vi "Agilent N6700 Series Data Log Voltage Sine Wave.vi"() -> ()   [LabVIEW 2018]
doc: "Configures the channel output range, waveform characteristics, sine wave, waveform trigger source, voltage trigger mode and enable output on a specified channel. This VI also configure the data logger, initiates data log, send a software trigger, configure data log markers and fetchs the peak to peak value of the data log.\n\n<b>Note:</b>\n\nThis VI only applies to the N6705B and N6705C DC Power Analyzer."
uses:
  Public/Configuration/Waveform/Configure Waveform (Sine Wave).vi
  <instrlib>/Agilent N6700 Series/Agilent N6700 Series.lvlib
panel:
  in  "Frequency (1.0 Hz)":dbl=1.0 format="%^.3e"
  in  "Data Log File Path":string="dlog example.dlog"
  in  "Voltage Range (5.0 V)":dbl=5.0 format="%^.3e"
  in  "Data Log Duration (15 s)":i32=15
  in  "Data Log Marker 2 (10.0 s)":dbl=10.0 format="%^.3e"
  in  "Data Log Marker 1 (7.5 s)":dbl=7.5 format="%^.3e"
  out "Peak to Peak Voltage":dbl format="%^.3e"
  in  "Channel Name (1)":string="1"
  in  "VISA resource name":refnum<visa-resource-name>
  # "(c) 2012-2019  National Instruments.  ALL RIGHTS RESERVED."
  # "Agilent N6705 DC Power Supply"
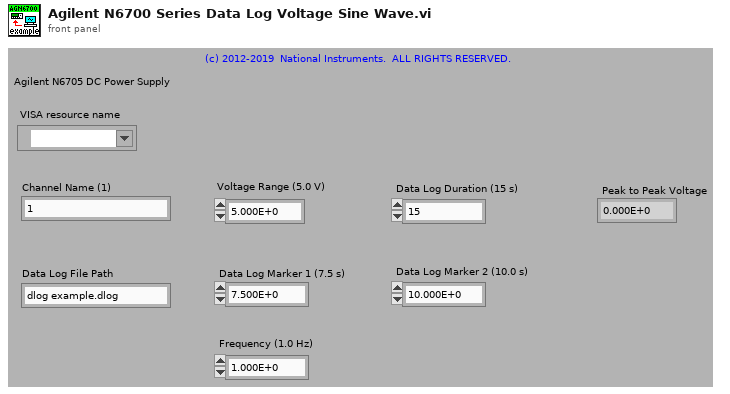
[diagram p1: front panel]
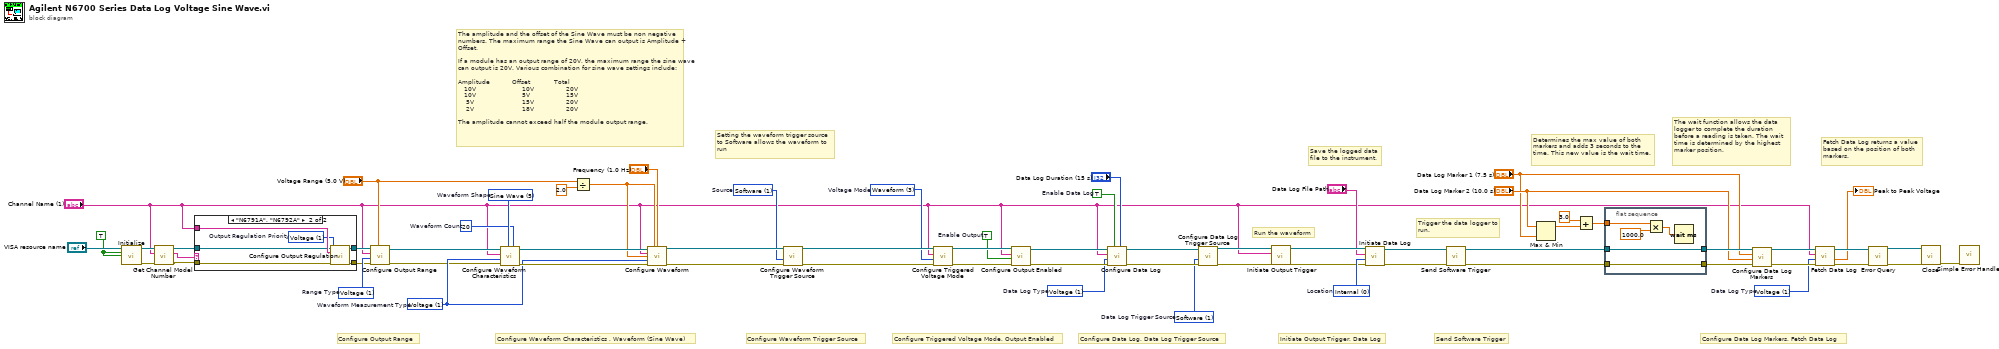
[diagram p0: block diagram]
diagram:
  w12 = 1 items=["Voltage"=1, "Current"=0]  # Data Log Type
  w25 = 20  # Waveform Count
  w26 = 1 items=["External", "Software", "Immediate", "Voltage1", "Voltage2", "Voltage3", "Voltage4", "Current1", "Current2", "Current3", "Current4"]  # Data Log Trigger Source
  w30 = 1 items=["Voltage"=1, "Current"=0]  # Range Type
  w37 = 3 items=["Fixed", "Step", "List", "Waveform"]  # Voltage Mode
  w11 = TRUE  # Enable Data Log
  w46 = TRUE  # Enable Output
  w51 = u16 1 items=["External", "Software", "Pin 1", "Pin 2", "Pin 3", "Transient 1", "Transient 2", "Transient 3", "Transient 4"]  # Source
  w38 = 1 items=["Voltage"=1, "Current"=0]  # Data Log Type
  w54 = TRUE ("Reset? (T: Yes)")
  w56 = 5 items=["None", "Constant Dwell", "Exponential", "Pulse", "Ramp", "Sine Wave", "Staircase", "Step", "Trapezoid", "Sequence", "User Defined"]  # Waveform Shape
  w57 = 0 items=["Internal", "External"]  # Location
  w58 = 1 items=["Voltage"=1, "Current"=0]  # Waveform Measurement Type
  # "Fetch Data Log returns a value\nbased on the position of both\nmarkers."
  # "Initiate Output Trigger, Data Log"
  # "Send Software Trigger"
  # "Configure Data Log Markers, Fetch Data Log"
  # "Configure Triggered Voltage Mode, Output Enabled"
  # "Configure Waveform Trigger Source"
  # "Run the waveform"
  # "Configure Output Range"
  # "Configure Data Log, Data Log Trigger Source"
  # "Configure Waveform Characteristics , Waveform (Sine Wave)"
  # "Determines the max value of both markers and adds 3 seconds to the time. This new value is the wait time."
  # "Trigger the data logger to run."
  # "Save the logged data\nfile to the instrument."
  # "Setting the waveform trigger source\nto Software allows the waveform to\nrun"
  # "The amplitude and the offset of the Sine Wave must be non negative numbers. The maximum range the Sine Wave can output is Amplitude + Offset.\n\nIf a module has an output range of 20V, the maximum range the sine wave can output is 20V. Various combination for sine wave settings include:\n\nAmplitude           Offset            Total\n   10V                       10V                20V\n   10V                       5V                  15V\n    5V                        15V                20V\n    2V                        18V                20V\n\nThe amplitude cannot exceed half the module output range."
  # "The wait function allows the data logger to complete the duration before a reading is taken. The wait\ntime is determined by the highest marker position."
  n1 = call "Initialize.vi"("VISA resource name"="VISA resource name", "ID Query? (T: Yes)"=w54, "Reset? (T: Yes)"=w54) -> ("VISA resource name out"=w6:refnum<visa-resource-name>, "error out"=w5:errorcluster)  [unwired: 11 in]
  n2 = call "Get Channel Model Number.vi"("error in (no error)"=w5, "Channel Name (1)"="Channel Name (1)", "VISA resource name"=w6) -> ("error out"=w4:errorcluster, "Model Number"=w2:string, "VISA resource name out"=w3:refnum<visa-resource-name>)  [unwired: 6 in]
  n3 = case shown="\"N6791A\", \"N6792A\"" w2 {
    tunnel: [w67 w73] -> w8
    tunnel: [w66 w72] -> w7
    tunnel: "Channel Name (1)" -> [_ w71]
    tunnel: w4 -> [w66 w68]
    tunnel: w3 -> [w67 w69]
    frame Default {
      # "The default priority for N679x is current."
    }
    frame "N6791A", "N6792A" {
      w70 = 1 items=["Voltage"=1, "Current"=0]  # Output Regulation Priority
      n4 = call "Configure Output Regulation.vi"("VISA resource name"=w69, "Channel Name (1)"=w71, "Output Regulation Priority (1: Voltage)"=w70, "error in (no error)"=w68) -> ("VISA resource name out"=w73:refnum<visa-resource-name>, "error out"=w72:errorcluster)  [unwired: 10 in]
    }
  }
  n5 = call "Configure Output Range.vi"("Range (0.0)"="Voltage Range (5.0 V)", "error in (no error)"=w7, "Range Type (1: Voltage)"=w30, "Channel Name (1)"="Channel Name (1)", "VISA resource name"=w8) -> ("error out"=w32:errorcluster, "VISA resource name out"=w31:refnum<visa-resource-name>)  [unwired: 5 in]
  n6 = call "Configure Waveform Characteristics.vi"("Waveform Count (1)"=w25, "Waveform Shape (0: None)"=w56, "error in (no error)"=w32, "Waveform Type (1: Voltage)"=w58, "Channel Name (1)"="Channel Name (1)", "VISA resource name"=w31) -> ("error out"=w59:errorcluster, "VISA resource name out"=w60:refnum<visa-resource-name>)  [unwired: 4 in]
  n7 = Divide(x="Voltage Range (5.0 V)", y=2.0) -> (x/y=w28:dbl)
  n8 = call-poly "Configure Waveform.vi"("VISA resource name"=w60, "Offset (0.0)"=w28, "Frequency (1.0 Hz)"="Frequency (1.0 Hz)", "Channel Name (1)"="Channel Name (1)", "Amplitude (0.0)"=w28, "Waveform Type (1: Voltage)"=w58, "error in (no error)"=w59) -> ("VISA resource name out"=w52:refnum<visa-resource-name>, "error out"=w53:errorcluster)  [unwired: 7 in]
  n9 = call "Configure Waveform Trigger Source.vi"("error in (no error)"=w53, "Source (2: Immediate)"=w51, "VISA resource name"=w52) -> ("error out"=w50:errorcluster, "VISA resource name out"=w49:refnum<visa-resource-name>)  [unwired: 7 in]
  n10 = call "Configure Triggered Voltage Mode.vi"("error in (no error)"=w50, "Voltage Mode (0: Fixed)"=w37, "Channel Name (1)"="Channel Name (1)", "VISA resource name"=w49) -> ("error out"=w47:errorcluster, "VISA resource name out"=w48:refnum<visa-resource-name>)  [unwired: 6 in]
  n11 = call "Configure Output Enabled.vi"("error in (no error)"=w47, "Enable Output (False)"=w46, "Channel Name (1)"="Channel Name (1)", "VISA resource name"=w48) -> ("error out"=w42:errorcluster, "VISA resource name out"=w41:refnum<visa-resource-name>)  [unwired: 6 in]
  n12 = call "Configure Data Log.vi"("Data Log Duration (30 s)"="Data Log Duration (15 s)", "Enable Data Log (True)"=w11, "error in (no error)"=w42, "Data Log Type (1: Voltage)"=w38, "Channel Name (1)"="Channel Name (1)", "VISA resource name"=w41) -> ("error out"=w39:errorcluster, "VISA resource name out"=w40:refnum<visa-resource-name>)  [unwired: 4 in]
  n13 = call "Configure Data Log Trigger Source.vi"("error in (no error)"=w39, "Data Log Trigger Source (2: Immediate)"=w26, "VISA resource name"=w40) -> ("error out"=w22:errorcluster, "VISA resource name out"=w24:refnum<visa-resource-name>)  [unwired: 7 in]
  n14 = call "Initiate Output Trigger.vi"("error in (no error)"=w22, "Channel Name (1)"="Channel Name (1)", "VISA resource name"=w24) -> ("error out"=w21:errorcluster, "VISA resource name out"=w23:refnum<visa-resource-name>)  [unwired: 7 in]
  n15 = call "Initiate Data Log.vi"("error in (no error)"=w21, "Location (0: Internal)"=w57, "Data Log File Path (data1.dlog)"="Data Log File Path", "VISA resource name"=w23) -> ("error out"=w35:errorcluster, "VISA resource name out"=w36:refnum<visa-resource-name>)  [unwired: 6 in]
  n16 = call "Send Software Trigger.vi"("error in (no error)"=w35, "VISA resource name"=w36) -> ("error out"=w34:errorcluster, "VISA resource name out"=w33:refnum<visa-resource-name>)  [unwired: 8 in]
  n17 = Max & Min(x="Data Log Marker 2 (10.0 s)", y="Data Log Marker 1 (7.5 s)") -> (max(x,y)=w16:dbl)  [unwired: 1 out]
  n18 = Add(x=3.0, y=w16) -> (x+y=w20:dbl)
  n19 = flat-sequence {
    tunnel: w34 -> [w78]
    tunnel: [w78] -> w17
    tunnel: w33 -> [w77]
    tunnel: [w77] -> w18
    tunnel: w20 -> [w76]
    frame #0 {
      n20 = Multiply(x=w76, y=1000.0) -> (x*y=w75:dbl)
      n21 = Wait (ms)(milliseconds to wait=w75) -> ()  [unwired: 1 out]
    }
  }
  n22 = call "Configure Data Log Markers.vi"("error in (no error)"=w17, "Data Log Marker 2 (27.5 s)"="Data Log Marker 2 (10.0 s)", "Data Log Marker 1 (7.5 s)"="Data Log Marker 1 (7.5 s)", "VISA resource name"=w18) -> ("error out"=w62:errorcluster, "VISA resource name out"=w61:refnum<visa-resource-name>)  [unwired: 6 in]
  n23 = call "Fetch Data Log.vi"("error in (no error)"=w62, "Data Log Type (1: Voltage)"=w12, "Channel Name (1)"="Channel Name (1)", "VISA resource name"=w61) -> ("error out"=w64:errorcluster, "Peak to Peak"=→"Peak to Peak Voltage":dbl, "VISA resource name out"=w65:refnum<visa-resource-name>)  [unwired: 5 in]
  n24 = call "Error Query.vi"("VISA resource name"=w65, "error in (no error)"=w64) -> ("VISA resource name out"=w43:refnum<visa-resource-name>, "error out"=w44:errorcluster)  [unwired: 10 in, 2 out]
  n25 = call "Close.vi"("VISA resource name"=w43, "error in (no error)"=w44) -> ("error out"=w45:errorcluster)  [unwired: 13 in]
  n26 = call <vilib>:"Simple Error Handler.vi"("error in (no error)"=w45) -> ()  [unwired: 4 in, 5 out]
